vi "calcErrorSD.vi"(3 "array of OD":dbl[][](array[numeric]), 4 "OD":dbl[](array[numeric]), 5 "Numeric in":i32) -> (0 "error out":dbl, 1 "average out":dbl[](array[numeric]), 2 "Array out":dbl[][](array[numeric]))   [LabVIEW 2015]
uses:
  <vilib>/Analysis/baseanly.llb/Mean (DBL).vi
  globalVarSD.vi
  <vilib>/Analysis/NI_AALBase.lvlib
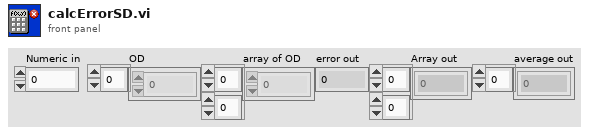
[diagram p1: front panel]
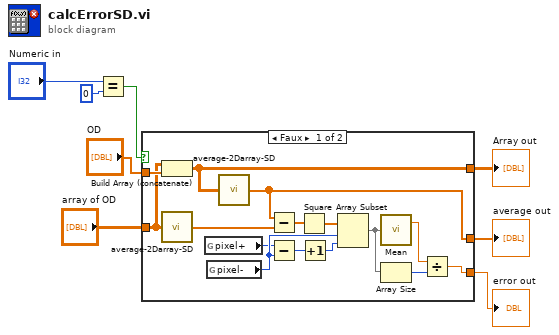
[diagram p0: block diagram]
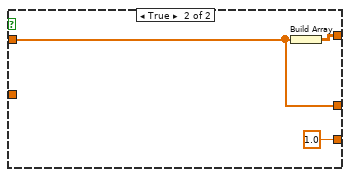
[diagram p2: hidden frame]
diagram:
  n1 = Equal?(x="Numeric in", y=0) -> (x = y?=w3:bool)
  n2 = case shown="Faux" w3 {
    tunnel: [w21 w26] -> w6
    tunnel: "OD" -> [w20 w24]
    tunnel: "array of OD" -> [w11 _]
    tunnel: [w19 1.0] -> w7
    tunnel: [w9 w24] -> w1
    frame False {
      n3 = Build Array (concatenate)(w11, w20) -> (w21:dbl[][])
      n4 = call "average-2Darray-SD.vi"("2D array"=w11) -> ("out array"=w10:dbl[])
      n5 = global read "globalVarSD.vi" "pixel+"() -> (w14:i32)
      n6 = global read "globalVarSD.vi" "pixel-"() -> (w16:i32)
      n7 = call "average-2Darray-SD.vi"("2D array"=w21) -> ("out array"=w9:dbl[])
      n8 = Subtract(x=w9, y=w10) -> (x-y=w22:dbl[])
      n9 = Subtract(x=w14, y=w16) -> (x-y=w17:i32)
      n10 = Square(x=w22) -> (x^2=w15:dbl[])
      n11 = Increment(x=w17) -> (x+1=w18:i32)
      n12 = Array Subset(array=w15, index=w16, length=w18) -> (w13:dbl[])
      n13 = call-poly <vilib>:"Mean.vi"("X"=w13) -> ("mean"=w23:dbl)  [unwired: 1 out]
      n14 = Array Size(array=w13) -> (size(s)=w12:i32)
      n15 = Divide(x=w23, y=w12) -> (x/y=w19:dbl)
    }
    frame True {
      n16 = Build Array(w24) -> (w26:dbl[][])
    }
  }
  "error out" <- w7
  "Array out" <- w6
  "average out" <- w1
